vi "from string.vi"(8 "error in":errorcluster, 9 "data":string, 10 "version":string, 11 "Instrument configuration":refnum<class "Instrument configuration.lvclass">) -> (0 "error out":errorcluster, 3 "Instrument configuration out":refnum<class "Instrument configuration.lvclass">)   [LabVIEW 2025, in "Abstract Engine.lvlib" / "Instrument configuration.lvclass"]
doc: "Provides an interface for loading a module configuration from a file or other serialized data source. It is recommended that all children of this class store data in two sets--data required for its own initialization, and any data required for parent initialization--and that each implementation uses the <b>Call Parent Method</b> primitive to de-serialize parent information.Copyright 2017 National Instruments Corporation\n\nLicensed under the Apache License, Version 2.0 (the \"License\"); you may not use this file except in compliance with the License. You may obtain a copy of the License at http://www.apache.org/licenses/LICENSE-2.0\nUnless required by applicable law or agreed to in writing, software distributed under the License is distributed on an \"AS IS\" BASIS, WITHOUT WARRANTIES OR CONDITIONS OF ANY KIND, either express or implied. See the License for the specific language governing permissions and limitations under the License."
uses:
  Instrument configuration.lvclass
  Instrument configuration.lvclass/Instrument configuration.ctl
  Users/Public/Documents/Sandia National Labs/TSS Plugin/CEF.lvlibp/serializable configuration/CEF_serializable configuration.lvclass
  Default Instrument.ctl
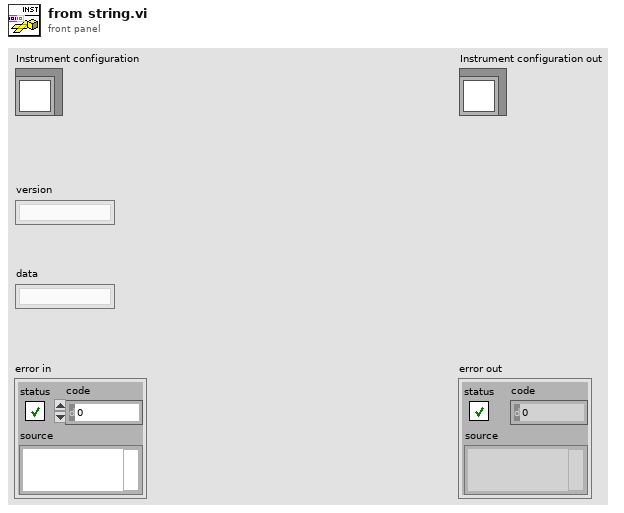
[diagram p1: front panel]
types:
  T1 = typedef "Abstract Engine.lvlib/Instrument configuration.lvclass/Default Instrument.ctl" = cluster{"Type":string, "Address":string, "SW Alias":string, "Description":string, "Enabled":bool}
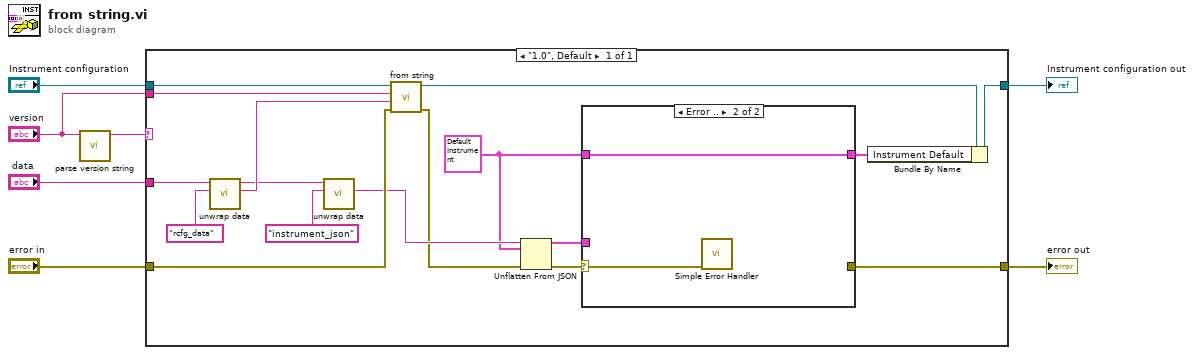
[diagram p0: block diagram]
diagram:
  n1 = call "parse version string.vi"("full version"="version") -> ("major.minor version"=w2:string)  [unwired: 7 in, 3 out]
  n2 = case shown="\"1.0\", Default" w2 {
    tunnel: "Instrument configuration" -> [w24]
    tunnel: [w16] -> w6
    tunnel: "data" -> [w22]
    tunnel: "error in" -> [w17]
    tunnel: [w10] -> w5
    tunnel: "version" -> [w13]
    frame "1.0", Default {
      w8 = T1 {"Type"="None", "Address"="localhost", "SW Alias"="Type = Class \n", "Description"="none", "Enabled"=TRUE} ("Default Engine")
      n3 = call "unwrap data.vi"("identifier"="rcfg_data" ("additional identifier"), "data to unwrap"=w22) -> ("unwrapped data"=w20:string, "remaining string"=w19:string)  [unwired: 8 in]
      n4 = call "unwrap data.vi"("identifier"="instrument_json" ("additional identifier"), "data to unwrap"=w19) -> ("unwrapped data"=w15:string)  [unwired: 8 in, 1 out]
      n5 = call-parent "from string.vi"("error in"=w17, "data"=w20, "version"=w13, "CEF_Configuration in"=w24) -> ("error out"=w14:errorcluster, "CEF_Configuration out"=w23:refnum<class "Instrument configuration.lvclass">)  [unwired: 6 in]
      n6 = Unflatten From JSON(JSON string=w15, type and defaults=w8, error in (no error)=w14) -> (value=w11:T1, error out=w12:errorcluster)  [unwired: 4 in]
      n7 = case shown="Error .." w12 {
        selector: w12 -> [w25 w27]
        tunnel: w11 -> [w26 _]
        tunnel: [w26 w28] -> w9
        tunnel: w8 -> [_ w28]
        tunnel: [w25 _] -> w10
        frame No Error {
        }
        frame Error {
          n8 = call <vilib>:"Simple Error Handler.vi"("error in (no error)"=w27) -> ()  [unwired: 4 in, 5 out]
        }
      }
      n9 = Bundle By Name(cluster=w23, "Instrument Default"=w9) -> (w16:refnum<class "Instrument configuration.lvclass">)
    }
  }
  "error out" <- w5
  "Instrument configuration out" <- w6
